vi "Group Delay Compensation.vi"() -> ()   [LabVIEW 2023]
doc: "Demonstrates how to use the DFD Group Delay Compensator VI to generate an infinite impulse response (IIR) filter that has the same magnitude response as the original filter. The new IIR filter contains an approximately constant group delay in the frequency ranges you specify.\n\nComplete the following steps to use this VI. \n1) Run the VI.\n2) Observe the Group Delay graph.\n3) Modify the filter specifications and run the VI again.\n4) Observe the Group Delays graph. Set the <B>Frequency Ranges</B> in which you want the group delay to be constant and run the VI again.\n5) Observe the Group Delays graph to see if the group delay in the specified frequency range is approximately constant.\n6) Observe the Magnitude Response of Compensator graph to verify the magnitude response equals 1.\n7) Modify the settings such as <B>Compensator Order</B>, <B>Frequency Ranges</B>, and <B>Integer Group Delay</B>, and run the VI again.\n8) Observe the Group Delays graph to view the result of the modifications.\n9) Examine the block diagram to learn how to use the DFD Group Delay Compensator VI."
uses:
  <vilib>/addons/Digital Filter Design/_Objects.llb/DFD Filter Frequence Specification (Design).ctl
  <vilib>/addons/Digital Filter Design/_Objects.llb/DFD Filter Ripple Specification (Design).ctl
  <vilib>/addons/Digital Filter Design/Analysis.llb/DFD Plot Freq Response (Linear-Spaced).vi
  <vilib>/addons/Digital Filter Design/NI_DigFilterLicensed.lvlib
panel:
  out "Error Message":string
  out "Magnitude Response of Compensator":cluster{"f0":dbl, "df":dbl, "values":dbl[]}[](graph)
  out "Group Delays":cluster{"f0":dbl, "df":dbl, "values":dbl[]}[](graph)
  in  "Integer Group Delay?":bool=TRUE
  in  "Frequency Ranges [Hz]":cluster{"low":dbl, "high":dbl}[](array[cluster])=[{"low"=0.0, "high"=200.0}]
  in  "Compensator Order":i32=6
  in  "Sampling Frequency [Hz]":dbl=1000.0 format="%.2f"
  in  "Ripple Specifications":T1={"passband"=0.1, "stopband"=60.0, "dB/linear? (T: dB)"=TRUE}
  in  "Frequency Sepcifications [Hz]":T2={"fpass 1"=200.0, "fstop 1"=300.0, "fpass 2 "=0.0, "fstop 2"=0.0}
  in  "Filter Type":T3(ring)
  in  "Design Method":T4(ring)=enum."Elliptic"
  # "Select Help>>Show Context Help and move the cursor over the VI icon for more information."
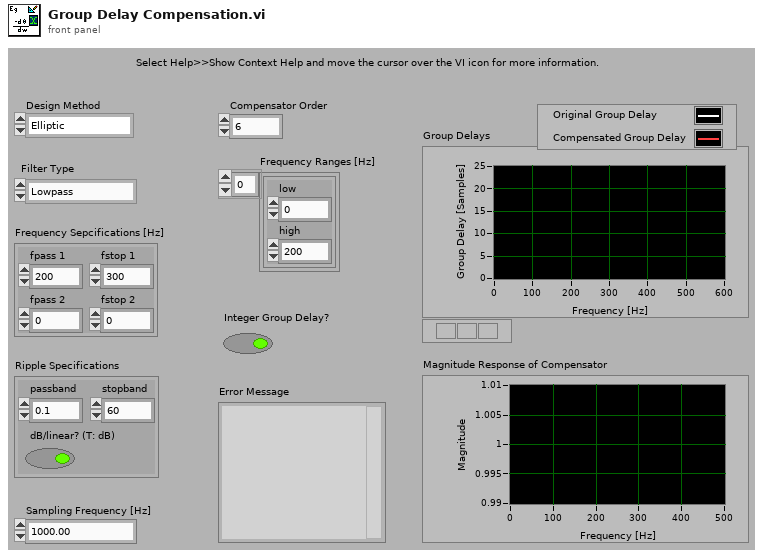
[diagram p1: front panel]
types:
  T1 = typedef "NI_DigFilterLicensed.lvlib/DFD Filter Ripple Specification (Design).ctl" = cluster{"passband":dbl, "stopband":dbl, "dB/linear? (T: dB)":bool}
  T2 = typedef "NI_DigFilterLicensed.lvlib/DFD Filter Frequence Specification (Design).ctl" = cluster{"fpass 1":dbl, "fstop 1":dbl, "fpass 2 ":dbl, "fstop 2":dbl}
  T3 = enum16{"Lowpass", "Highpass", "Bandpass", "Bandstop"}
  T4 = enum16{"Butterworth", "Chebyshev", "Inverse Chebyshev", "Elliptic"}
  T5 = typedef "NI_DigFilterLicensed.lvlib/DFD Filter Obj.ctl" = cluster{"mSRate_Fs":dbl, "mSRate_Version":string, "mSRate_Comments":string, "mSRate_OrgCoef":T6, "mSRate_CurCoef":T6, "mSRate_Quantized?":bool, "mSRate_QCoef":T6, "mSRate_QSettings":T8[], "mSRate_Order":i32, "mSRate_Scaling":cluster{"mSRate_ScaleByPowerOf2?":bool, "mSRate_ScaleType":T10}}
  T6 = typedef "NI_DigFilterLicensed.lvlib/DFD Filter Coef.ctl" = cluster{"type":T7, "gain":dbl, "coef a (k)":dbl[], "coef b (v)":dbl[]}
  T7 = typedef "NI_DigFilterLicensed.lvlib/DFD Filter Structure Type Selector.ctl" = enum16{"Undefined", "FIR Direct Form", "FIR Direct Form Transposed", "FIR Symmetric", "FIR Antisymmetric", "IIR Direct Form I", "IIR Direct Form I Transposed", "IIR Direct Form II", "IIR Direct Form II Transposed", "IIR Cascaded Second Order Sections Form I", "IIR Cascaded Second Order Sections Form I Transposed", "IIR Cascaded Second Order Sections Form II", "IIR Cascaded Second Order Sections Form II Transposed", "Lattice Allpass (basic sections)", "Lattice Allpass (one multiplier sections)", "Lattice Allpass (normalized sections)", "Lattice AR (basic sections)", "Lattice AR (one multiplier sections)", "Lattice AR (normalized sections)", "Lattice MA (minimum phase)", "Lattice MA (maximum phase)", "Lattice ARMA (basic sections)", "Lattice ARMA (one multiplier sections)", "Lattice ARMA (normalized sections)"}
  T8 = typedef "NI_DigFilterLicensed.lvlib/dfd_Internal Quantization Settings.ctl" = cluster{"source":T9, "wl":i16, "iwl":i16, "overflow mode":enum16{"Saturation", "Wrap"}, "rounding mode":enum16{"Nearest", "Truncation"}, "signed?":bool}
  T9 = typedef "NI_DigFilterLicensed.lvlib/dfd_Internal Quantization Srcs.ctl" = u16
  T10 = typedef "NI_DigFilterLicensed.lvlib/DFD Coef Norm Type.ctl" = enum16{"No Norm", "Time Domain 1-Norm", "Time Domain 2-Norm", "Time Domain Inf-Norm"}
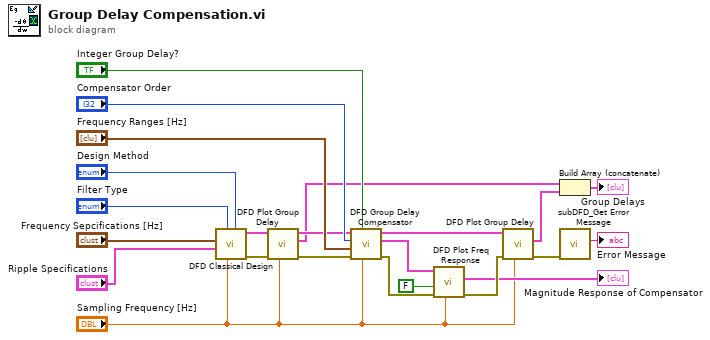
[diagram p0: block diagram]
diagram:
  n1 = call <vilib>:"DFD Classical Design.vi"("design method"="Design Method", "fs [Hz]"="Sampling Frequency [Hz]", "filter type"="Filter Type", "ripple specs"="Ripple Specifications", "freq specs [Hz]"="Frequency Sepcifications [Hz]") -> ("error out"=w12:errorcluster, "filter out"=w13:T5)  [unwired: 1 in, 4 out]
  n2 = call <vilib>:"DFD Plot Group Delay.vi"("fs [Hz]"="Sampling Frequency [Hz]", "error in (no error)"=w12, "filter in"=w13) -> ("error out"=w10:errorcluster, "group delay"=w9:cluster{"f0":dbl, "df":dbl, "values":dbl[]}[], "filter out"=w11:T5)  [unwired: 1 in, 5 out]
  n3 = call <vilib>:"DFD Group Delay Compensator.vi"("fs [Hz]"="Sampling Frequency [Hz]", "integer group delay?"="Integer Group Delay?", "error in (no error)"=w10, "freq ranges [Hz]"="Frequency Ranges [Hz]", "compensator order"="Compensator Order", "filter in"=w11) -> ("error out"=w7:errorcluster, "compensator"=w8:T5, "compensated filter"=w16:T5)  [unwired: 1 in, 2 out]
  n4 = call-poly <vilib>:"DFD Plot Freq Response.vi"("fs [Hz]"="Sampling Frequency [Hz]", "error in (no error)"=w7, "dB on? (T)"=FALSE, "filter in"=w8) -> ("error out"=w6:errorcluster, "magnitude response"=→"Magnitude Response of Compensator":cluster{"f0":dbl, "df":dbl, "values":dbl[]}[])  [unwired: 4 in, 2 out]
  n5 = call <vilib>:"DFD Plot Group Delay.vi"("fs [Hz]"="Sampling Frequency [Hz]", "error in (no error)"=w6, "filter in"=w16) -> ("error out"=w1:errorcluster, "group delay"=w15:cluster{"f0":dbl, "df":dbl, "values":dbl[]}[])  [unwired: 1 in, 6 out]
  n6 = Build Array (concatenate)(w9, w15) -> (→"Group Delays":cluster{"f0":dbl, "df":dbl, "values":dbl[]}[])
  n7 = call <vilib>:"subDFD_Get Error Message.vi"("error in (no error)"=w1) -> ("Error Message"=→"Error Message":string)  [unwired: 10 out]
